vi "Get Request Type.vi"(8 "error in (no error)":errorcluster, 11 "Sleep in":refnum<class "Sleep.lvclass">) -> (0 "error out":errorcluster, 2 "Request Type":string, 3 "Sleep out":refnum<class "Sleep.lvclass">)   [LabVIEW 2022 SP3, in "obs-websocket-lv.lvlib" / "Sleep.lvclass"]
uses:
  Sleep.lvclass
  Sleep.lvclass/Sleep.ctl
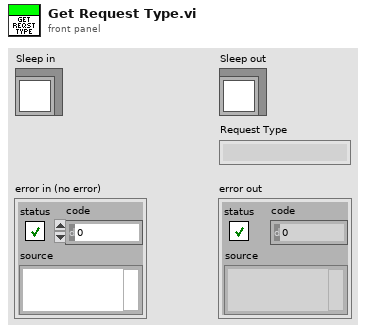
[diagram p1: front panel]
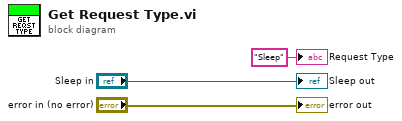
[diagram p0: block diagram]
diagram:
  "error out" <- "error in (no error)"
  "Sleep out" <- "Sleep in"
  "Request Type" <- "Sleep" ("Request Type")
